vi "Connect.vi"(8 "error in (no error)":errorcluster, 9 "Output Name":string, 10 "Input Name":string, 11 "Mux in":refnum<class "Mux.lvclass">) -> (0 "error out":errorcluster, 3 "Mux out":refnum<class "Mux.lvclass">)   [LabVIEW 2022 SP3]
uses:
  Mux.lvclass
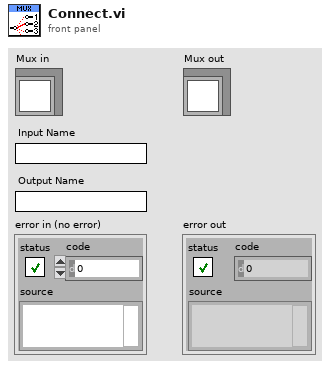
[diagram p1: front panel]
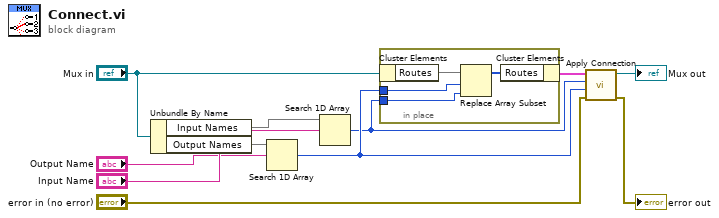
[diagram p0: block diagram]
diagram:
  n1 = Unbundle By Name("Mux in") -> ("Input Names"=w10, "Output Names"=w8)
  n2 = Search 1D Array(1D array=w8, element="Output Name") -> (index of element=w4:i32)  [unwired: 1 in]
  n3 = Search 1D Array(1D array=w10, element="Input Name") -> (index of element=w3:i32)  [unwired: 1 in]
  n4 = in-place {
    in-place-border: w4 -> [w14]
    in-place-border: w3 -> [w13]
    n5 = in-place-cluster #1("Mux in") -> ("Routes"=w15)
    n6 = Replace Array Subset(array=w15, new element=w13, index=w14) -> (w12:i32[])
    n7 = in-place-cluster #1("Routes"=w12) -> (w6:cluster{})
  }
  n8 = call-dynamic "Apply Connection.vi"("error in (no error)"="error in (no error)", "Output Index"=w4, "Input Index"=w3, "Mux in"=w6) -> ("error out"=→"error out":errorcluster, "Mux out"=→"Mux out":refnum<class "Mux.lvclass">)  [unwired: 6 in]
